vi "Create New File Name.vi"(1 "File Extension":string="txt", 2 "Path":path=path "C:/Users/pursley/Documents/Experiment Data") -> (0 "Path Out":path)   [LabVIEW 2017, in "HostCode.lvlib"]
uses:
  HostCode/HostCode.lvlib
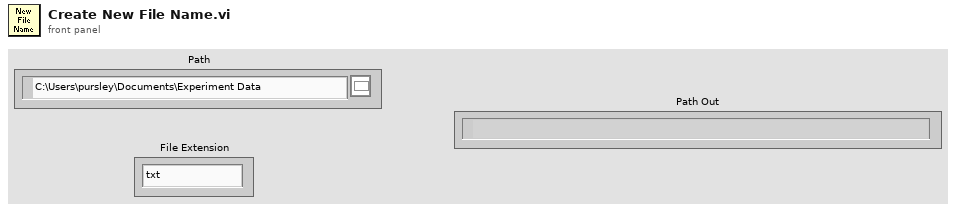
[diagram p1: front panel]
types:
  T1 = typedef "LVDateTimeRec.ctl" = cluster{"fractional second":dbl, "second":i32, "minute":i32, "hour":i32, "day of month":i32, "month":i32, "year":i32, "day of week":i32, "day of year":i32, "DST":i32}
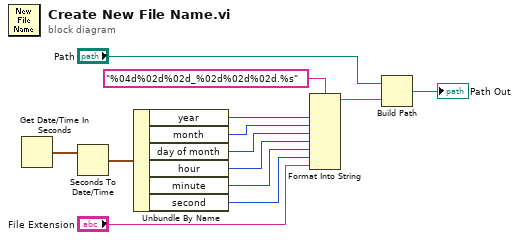
[diagram p0: block diagram]
diagram:
  n1 = Get Date/Time In Seconds() -> (seconds since 1Jan1904=w13:timestamp)
  n2 = Seconds To Date/Time(time stamp (now)=w13) -> (date time rec=w12:T1)  [unwired: 1 in]
  n3 = Unbundle By Name(w12) -> ("year"=w11:i32, "month"=w10:i32, "day of month"=w9:i32, "hour"=w8:i32, "minute"=w7:i32, "second"=w6:i32)
  n4 = Format Into String(format string="%04d%02d%02d_%02d%02d%02d.%s", w11, w10, w9, w8, w7, w6, "File Extension") -> (resulting string=w3:string)  [unwired: 2 in, 1 out]
  n5 = Build Path(base path="Path", name or relative path=w3) -> (appended path=→"Path Out":path)
